vi "GetDateTimeString.vi"() -> ()   [LabVIEW 2019]
panel:
  out "time string":string
  out "date string":string
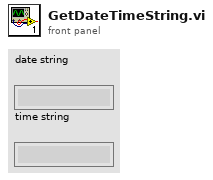
[diagram p1: front panel]
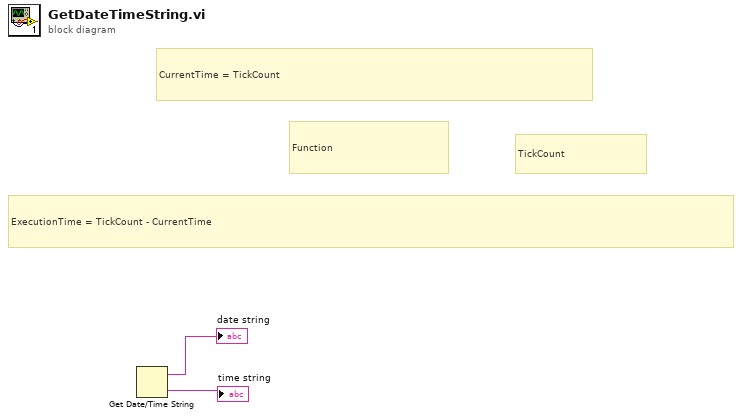
[diagram p0: block diagram]
diagram:
  # "TickCount"
  # "ExecutionTime = TickCount - CurrentTime"
  # "CurrentTime = TickCount"
  # "Function"
  n1 = Get Date/Time String() -> (date string=→"date string":string, time string=→"time string":string)  [unwired: 3 in]
